vi "DAQListUpdate.vi"(7 "Comm":T1, 8 "error in (no error)":errorcluster, 9 "ColNumbers":i32, 10 "Channels info":string[](array[string])=["燃烧室压力1\n[MPa]", "燃烧室压力1\n[MPa]"], 11 "List* in":refnum<vi>) -> (0 "error out":errorcluster, 2 "CHTag[]":string[](array[string]), 3 "List* out":refnum<vi>)   [LabVIEW 2016]
uses:
  Controls/DAQListOperation.ctl
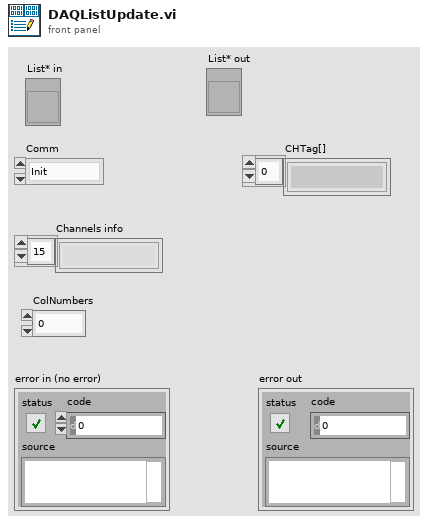
[diagram p1: front panel]
types:
  T1 = typedef "DAQListOperation.ctl" = enum16{"Init", "Clear", "Update Data", "Update CH Name", "Set List Property", "Get CHTag[]"}
  T2 = typedef "Global para Config.ctl" = cluster{"连续存储设置":cluster{"Save Mode":i32, "Sel Save Mode":i32, "FolderPath":path, "Filename":string, "Explation":string, "AutoPoint":i32, "Template":path}, "Latest Prj":path, "Tdms Ref*":refnum<k34>, "默认波形图个数":u8, "列表列数":u8}
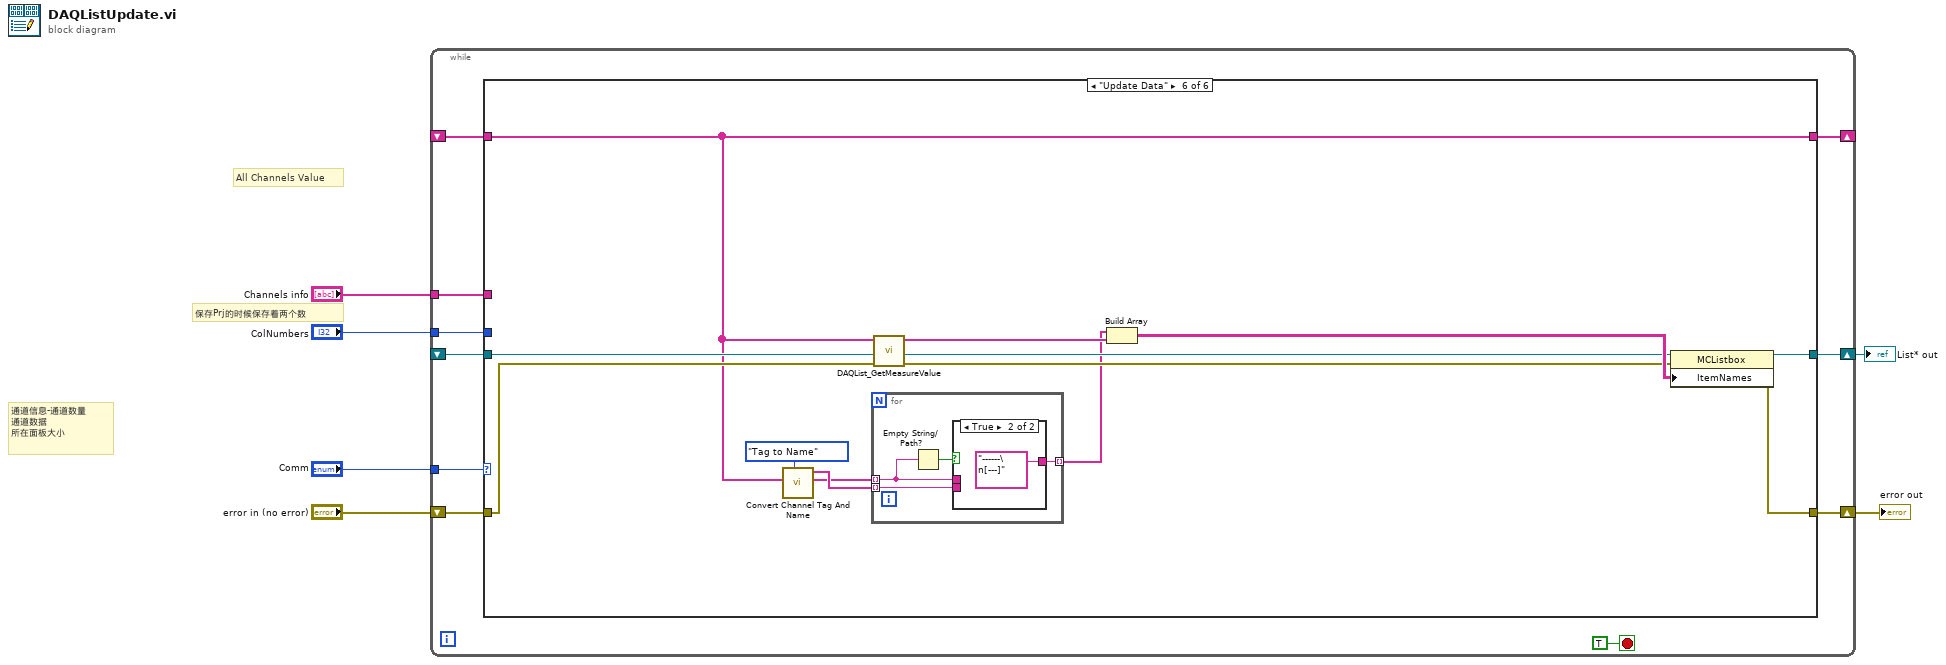
[diagram p0: block diagram]
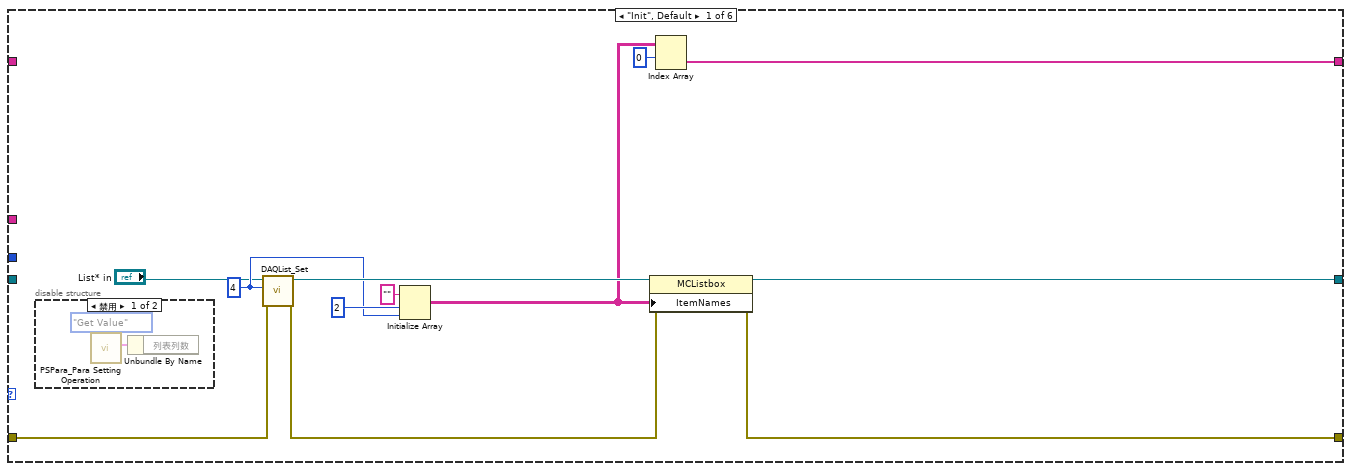
[diagram p2: hidden frame]
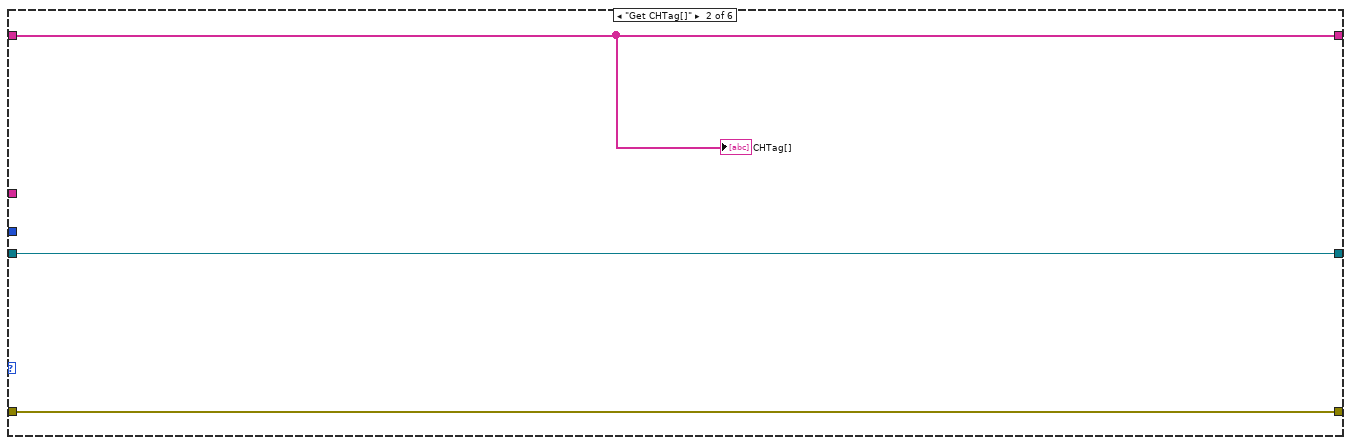
[diagram p4: hidden frame]
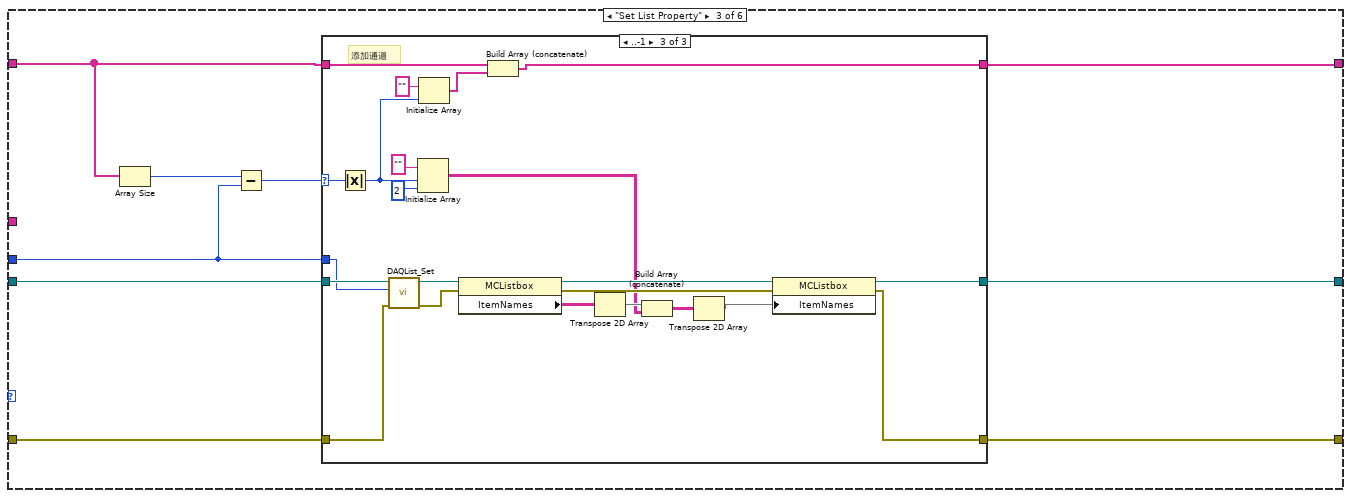
[diagram p5: hidden frame]
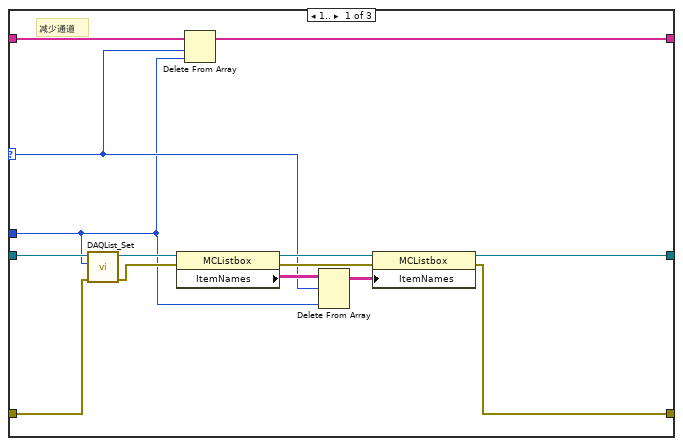
[diagram p6: hidden frame]
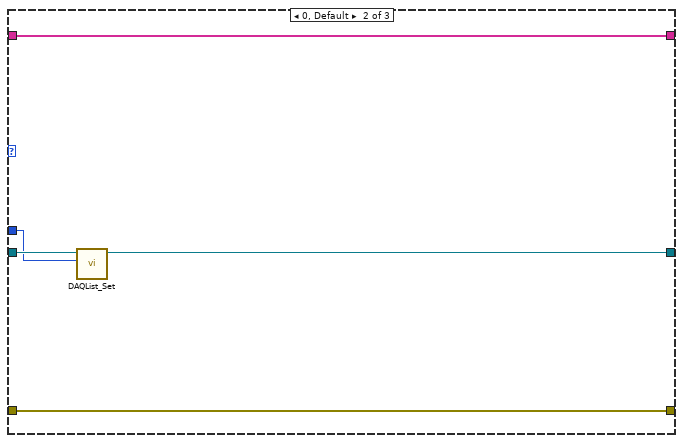
[diagram p7: hidden frame]
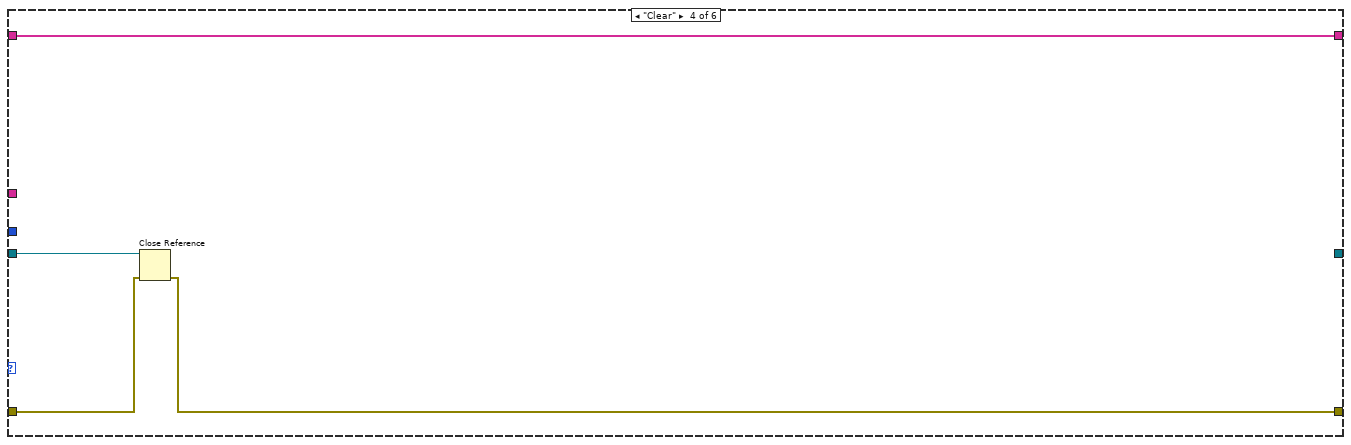
[diagram p8: hidden frame]
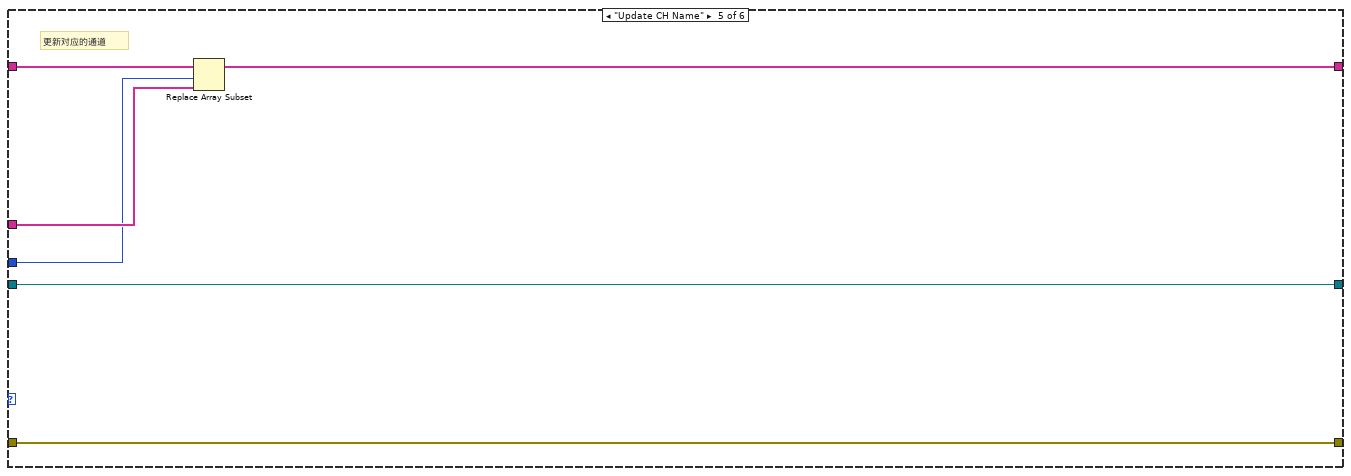
[diagram p9: hidden frame]
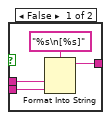
[diagram p10: hidden frame]
diagram:
  # "保存Prj的时候保存着两个数"
  # "All Channels Value"
  # "通道信息-通道数量\n通道数据\n所在面板大小"
  n1 = while {
    tunnel: "Comm" -> [w15]
    shift-right: [w12] -> w1
    shift-left: _ -> [w11]
    shift-right: [w13] -> w4
    shift-left: "error in (no error)" -> [w14]
    tunnel: "Channels info" -> [w10]
    tunnel: "ColNumbers" -> [w9]
    shift-right: [w7] -> _
    shift-left: _ -> [w8]
    stop <- TRUE stop-if-true
    n2 = case shown="\"Update Data\"" w15 {
      tunnel: w14 -> [w25 w33 w39 w87 w90 w99]
      tunnel: [w28 w33 w38 w86 w90 w104] -> w13
      tunnel: [w26 w32 w40 _ w89 w105] -> w12
      tunnel: w11 -> [_ w32 w41 w85 w89 w101]
      tunnel: w10 -> [_ _ _ _ w93 _]
      tunnel: w9 -> [_ _ w37 _ w91 _]
      tunnel: w8 -> [_ w31 w35 w84 w92 w94]
      tunnel: [w17 w31 w34 w84 w88 w94] -> w7
      frame "Init", Default {
        w21 = 4 ("dimension size")
        n3 = disable-structure shown="禁用" {
          frame Disabled {
            n4 = call "PSPara_Para Setting Operation.vi"("Operation"=enum16{"Set Value", "Get Value", "Initialize"}."Get Value") -> ("_Para"=w29:T2)  [unwired: 9 in, 1 out]
            n5 = Unbundle By Name(w29) -> ()  [unwired: 1 out]
          }
          frame Enabled {
          }
        }
        n6 = call "DAQList_Set.vi"("error in (no error)"=w25, "ColNumbers"=w21, "MulticolumnListbox in"="List* in") -> ("error out"=w24:errorcluster, "MulticolumnListbox out"=w23:refnum<vi>)  [unwired: 7 in]
        n7 = Initialize Array("", 2 ("dimension size"), w21) -> (w19:string[][])
        n8 = property class="MCListbox"(reference=w23, error in=w24, "ItemNames"=w19) -> (reference out=w26:refnum<vi>, error out=w28:errorcluster)
        n9 = Index Array(array=w19, index (row)=0 ("索引 (行)")) -> (element=w17:string[])  [unwired: 1 in]
      }
      frame "Get CHTag[]" {
        "CHTag[]" <- w31
      }
      frame "Set List Property" {
        n10 = Array Size(array=w35) -> (size(s)=w36:i32)
        n11 = Subtract(x=w36, y=w37) -> (x-y=w42:i32)
        n12 = case shown="..-1" w42 {
          selector: w42 -> [w45 _ w83]
          tunnel: w41 -> [w56 w60 w80]
          tunnel: [w55 w59 w79] -> w40
          tunnel: w39 -> [w53 w61 w78]
          tunnel: [w54 w61 w77] -> w38
          tunnel: w37 -> [w44 w58 w76]
          tunnel: w35 -> [w46 w57 w63]
          tunnel: [w43 w57 w62] -> w34
          frame 1.. {
            # "减少通道"
            n13 = call "DAQList_Set.vi"("error in (no error)"=w53, "ColNumbers"=w44, "MulticolumnListbox in"=w56) -> ("error out"=w50:errorcluster, "MulticolumnListbox out"=w51:refnum<vi>)  [unwired: 7 in]
            n14 = property class="MCListbox"(reference=w51, error in=w50) -> (reference out=w49:refnum<vi>, error out=w48:errorcluster, "ItemNames"=w52:string[][])
            n15 = Delete From Array(array=w46, length=w45, index=w44) -> (array with subset deleted=w43:string[])  [unwired: 1 out]
            n16 = Delete From Array(array=w52, length=w45, index (col)=w44) -> (array with subset deleted=w47:string[][])  [unwired: 1 in, 1 out]
            n17 = property class="MCListbox"(reference=w49, error in=w48, "ItemNames"=w47) -> (reference out=w55:refnum<vi>, error out=w54:errorcluster)
          }
          frame 0, Default {
            n18 = call "DAQList_Set.vi"("ColNumbers"=w58, "MulticolumnListbox in"=w60) -> ("MulticolumnListbox out"=w59:refnum<vi>)  [unwired: 8 in, 1 out]
          }
          frame ..-1 {
            # "添加通道"
            n19 = Absolute Value(x=w83) -> (abs(x)=w65:i32)
            n20 = call "DAQList_Set.vi"("error in (no error)"=w78, "ColNumbers"=w76, "MulticolumnListbox in"=w80) -> ("error out"=w74:errorcluster, "MulticolumnListbox out"=w75:refnum<vi>)  [unwired: 7 in]
            n21 = Initialize Array("", w65, 2 ("dimension size")) -> (w67:string[][])
            n22 = Initialize Array("" ("元素"), w65) -> (w64:string[])
            n23 = property class="MCListbox"(reference=w75, error in=w74) -> (reference out=w68:refnum<vi>, error out=w73:errorcluster, "ItemNames"=w70:string[][])
            n24 = Build Array (concatenate)(w63, w64) -> (w62:string[])
            n25 = Transpose 2D Array(2D array=w70) -> (transposed array=w72:string[][])
            n26 = Build Array (concatenate)(w72, w67) -> (w71:string[][])
            n27 = Transpose 2D Array(2D array=w71) -> (transposed array=w69:string[][])
            n28 = property class="MCListbox"(reference=w68, error in=w73, "ItemNames"=w69) -> (reference out=w79:refnum<vi>, error out=w77:errorcluster)
          }
        }
      }
      frame "Clear" {
        n29 = Close Reference(reference=w85, error in (no error)=w87) -> (error out=w86:errorcluster)
      }
      frame "Update CH Name" {
        # "更新对应的通道"
        n30 = Replace Array Subset(array=w92, new element=w93, index=w91) -> (w88:string[])
      }
      frame "Update Data" {
        n31 = call "Convert Channel Tag And Name.vi"("Direction"=enum16{"Tag to Name", "Name to Tag"}."Tag to Name", "String[] in"=w94) -> ("String[] out"=w96:string[], "Unit[]"=w97:string[])  [unwired: 8 in]
        n32 = for {
          tunnel: w97 -> [w109] mode=indexing
          tunnel: w96 -> [w107] mode=indexing
          tunnel: [w106] -> w95 mode=indexing
          n33 = Empty String/Path?(string/path=w107) -> (empty?=w108:bool)
          n34 = case shown="True" w108 {
            tunnel: [w112 "------\n[---]"] -> w106
            tunnel: w107 -> [w111 _]
            tunnel: w109 -> [w110 _]
            frame False {
              n35 = Format Into String(format string="%s\n[%s]" ("格式字符串"), w111, w110) -> (resulting string=w112:string)  [unwired: 2 in, 1 out]
            }
            frame True {
            }
          }
        }
        n36 = call "DAQList_GetMeasureValue.vi"("error in (no error)"=w99, "Channel Tag[]"=w94) -> ("error out"=w98:errorcluster, "Channels Value"=w103:string[])  [unwired: 8 in]
        n37 = Build Array(w95, w103) -> (w102:string[][])
        n38 = property class="MCListbox"(reference=w101, error in=w98, "ItemNames"=w102) -> (reference out=w105:refnum<vi>, error out=w104:errorcluster)
      }
    }
  }
  "error out" <- w4
  "List* out" <- w1
